vi "Globals.vi"() -> ()   [LabVIEW 2014]
panel:
  in  "Connect":dbl
  in  "Direction":dbl
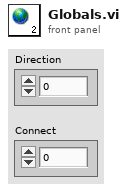
[diagram p1: front panel]
diagram:
